vi "macro_Analog_Delay.vi"   [LabVIEW 2019, in "Trajectory_Library.lvlib"]
uses:
  Trajectory_Library.lvlib
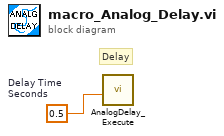
[diagram p0: block diagram]
diagram:
  w1 = 0.5  # Delay Time Seconds
  # "Delay"
  n1 = call "AnalogDelay_Execute.vi"("Delay Time"=w1) -> ()  [unwired: 9 in, 2 out]
